vi "Timeout Margin.vi"() -> (3 "y":dbl)   [LabVIEW 2012]
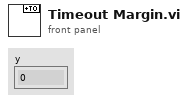
[diagram p1: front panel]
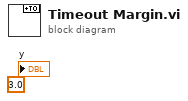
[diagram p0: block diagram]
diagram:
  "y" <- 3.0 ("y")
